vi "Mapping Init Loops v10.6.0.vi"(0 "Z Position":dbl, 1 "Mapping Params":T1 {"Step Size" min=0.1 max=30.0 step=0.1 format="%.1f"; "Y Stop Position" min=0.0 max=30.0 step=0.1 format="%.1f"; "Y Start Position" min=0.0 max=30.0 step=0.1 format="%.1f"; "X Stop Position" min=0.0 max=30.0 step=0.1 format="%.1f"; "X Start Position" min=0.0 max=30.0 step=0.1 format="%.1f"}) -> (2 "Start Positions":T2 {"Drive Z Position" min=-273.0 max=300000.0 step=0.0001 format="%.3f"; "Drive Y Position" min=-273.0 max=300000.0 step=0.0001 format="%.3f"; "Drive X Position" min=-273.0 max=300000.0 step=0.0001 format="%.3f"}, 3 "Step Size":dbl, 4 "X Steps":dbl, 5 "Y Steps":dbl)   [LabVIEW 2010]
uses:
  NPC3SG/TypeDefs/NPC3SG Current Values.ctl
  TypeDefs/Mapping Drive Params.ctl
  NPC3SG/TypeDefs/NPC3SG Set Positions.ctl
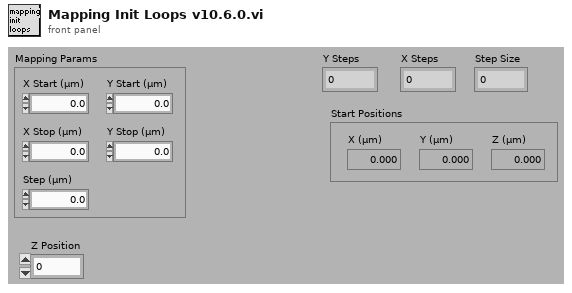
[diagram p1: front panel]
types:
  T1 = typedef "Mapping Drive Params.ctl" = cluster{"X Start Position":dbl, "X Stop Position":dbl, "Y Start Position":dbl, "Y Stop Position":dbl, "Step Size":dbl}
  T2 = typedef "NPC3SG Current Values.ctl" = cluster{"Drive X Position":dbl, "Drive Y Position":dbl, "Drive Z Position":dbl}
  T3 = typedef "NPC3SG Set Positions.ctl" = cluster{"Drive X Set":dbl, "Drive Y Set":dbl, "Drive Z Set":dbl}
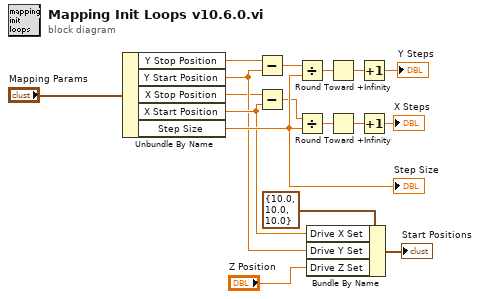
[diagram p0: block diagram]
diagram:
  n1 = Unbundle By Name("Mapping Params") -> ("Y Stop Position"=w7:dbl, "Y Start Position"=w10:dbl, "X Stop Position"=w8:dbl, "X Start Position"=w12:dbl, "Step Size"=w16:dbl)
  "Step Size" <- w16
  n2 = Subtract(x=w7, y=w10) -> (x-y=w1:dbl)
  n3 = Subtract(x=w8, y=w12) -> (x-y=w4:dbl)
  n4 = Divide(x=w1, y=w16) -> (x/y=w2:dbl)
  n5 = Divide(x=w4, y=w16) -> (x/y=w5:dbl)
  n6 = Bundle By Name(cluster=T3 {"Drive X Set"=10.0, "Drive Y Set"=10.0, "Drive Z Set"=10.0} ("Drive New Abs. Positions"), "Drive X Set"=w12, "Drive Y Set"=w10, "Drive Z Set"="Z Position") -> (→"Start Positions":T3)
  n7 = Round Toward +Infinity(x=w2) -> (ceil(x): smallest int >= x=w3:dbl)
  n8 = Round Toward +Infinity(x=w5) -> (ceil(x): smallest int >= x=w6:dbl)
  n9 = Increment(x=w3) -> (x+1=→"Y Steps":dbl)
  n10 = Increment(x=w6) -> (x+1=→"X Steps":dbl)
